vi "HandleObservationSync_003.vi"(8 "error in (no error)":errorcluster, 11 "S4GUI in":refnum<class "S4GUI.lvclass">) -> (0 "error out":errorcluster, 3 "S4GUI out":refnum<class "S4GUI.lvclass">)   [LabVIEW 2018, in "S4GUI.lvclass"]
uses:
  S4GUI.lvclass
  S4GUI.lvclass/S4GUI.ctl
  Instrument/Instrument.lvclass/Instrument.ctl
  Device/Optics/Optics.lvclass/Optics.ctl
  Server/Server.lvclass/Server.ctl
  Interface/Interface.lvclass/Interface.ctl
  Device/Optics/Opt_Selector/Opt_Selector.lvclass
  C:/Users/devstaff/sparc4/s4gui/Versao ZeroMQ REQ-REP/SPARC4_GUI -20241016_20241016/Device/Optics/Optics.lvclass
  Acquisition/Acquisition.lvclass
  C:/Users/devstaff/sparc4/s4gui/Versao ZeroMQ REQ-REP/SPARC4_GUI -20241016_20241016/Server/Server.lvclass
  SyncBox/Sync Box.lvclass
  Instrument/Instrument.lvclass
  Device/Optics/Opt_Continuous/Opt_Continuous.lvclass
  StateMachine/State Machine.lvclass
  Trigger/Trigger.lvclass
  Channel/Channel.lvclass
  Interface/Interface.lvclass
  TelFocus/TelFocus.lvclass
  SecMirror/SecMirror.lvclass
  Device/Optics/Optics.lvclass
  Server/Server.lvclass
panel:
  out "time1 3":u32
  out "time307":u32
  out "time9":u32
  out "time 10":u32
  out "delay 89":u32
  out "time1 2":u32
  out "delay Acq 2":u32
  out "time 8":u32
  out "delay 78":u32
  out "time elapsed 2":u32
  out "time7":u32
  out "time6":u32
  out "time5":u32
  out "time elapsed":u32
  out "timer351":u32
  out "delay wp 2":u32
  out "timer350":u32
  out "delay Acq":u32
  out "time308":u32
  out "delay wp":u32
  out "delay 3-4":u32
  out "time4":u32
  out "time3":u32
  out "time 2":u32
  out "time1":u32
  # "WAVEPLATE DURATION"
  # "ACS SETUP"
  # "Waveplate Test"
  # "Focus sequence"
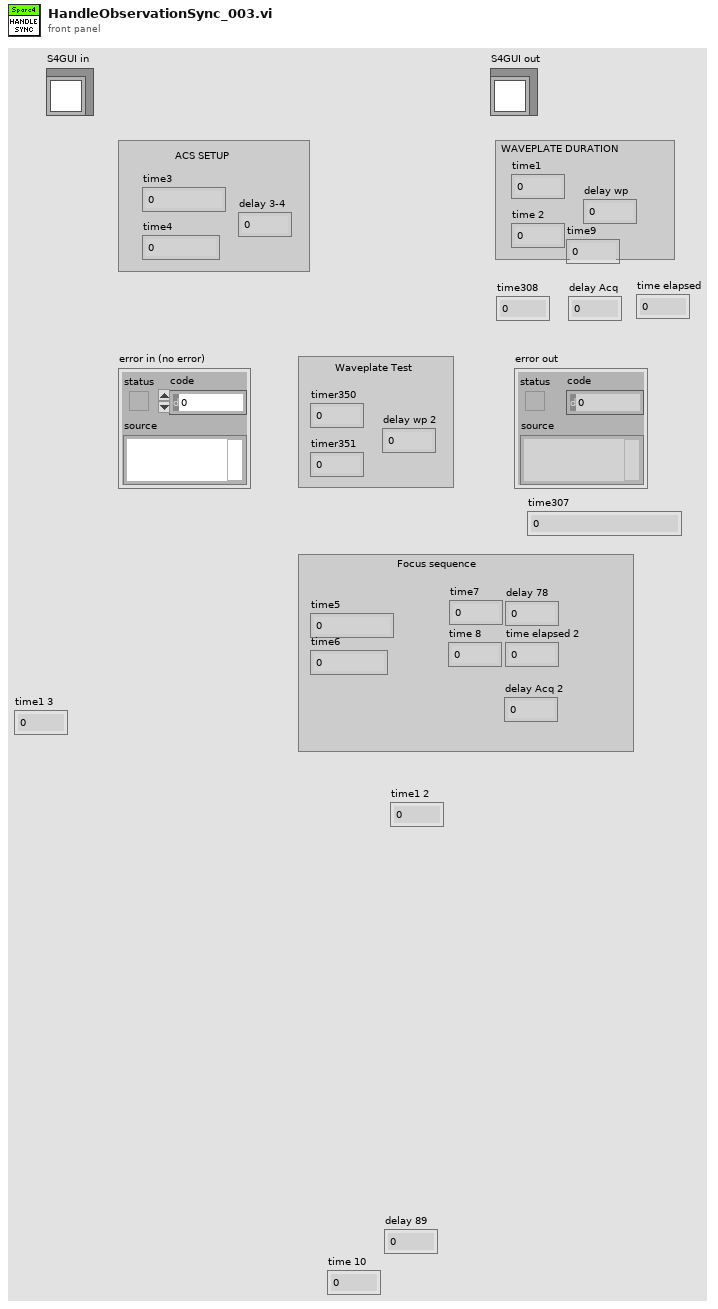
[diagram p1: front panel]
types:
  T1 = cluster{"ACQUISITION_MODE":u8, "TRIGGER_MODE":u8, "READ_MODE":u8, "PREAMP":u8, "READOUT_RATE":u8, "VERTICAL_SHIFT_SPEED":u8, "EM_MODE":u8, "EM_GAIN":u16, "SHUTTER_MODE":u8, "SHUTTER_TTL":u8, "SHUTTER_OPENING_TIME":u16, "SHUTTER_CLOSING_TIME":u16, "VBIN":u16, "HBIN":u16, "INITIAL_LINE":u16, "INITIAL_COLUMN":u16, "FINAL_LINE":u16, "FINAL_COLUMN":u16, "FRAME_TRANSFER":bool, "VERTICAL_CLOCK_VOLTAGE":u8, "AD_CHANNEL":u32}
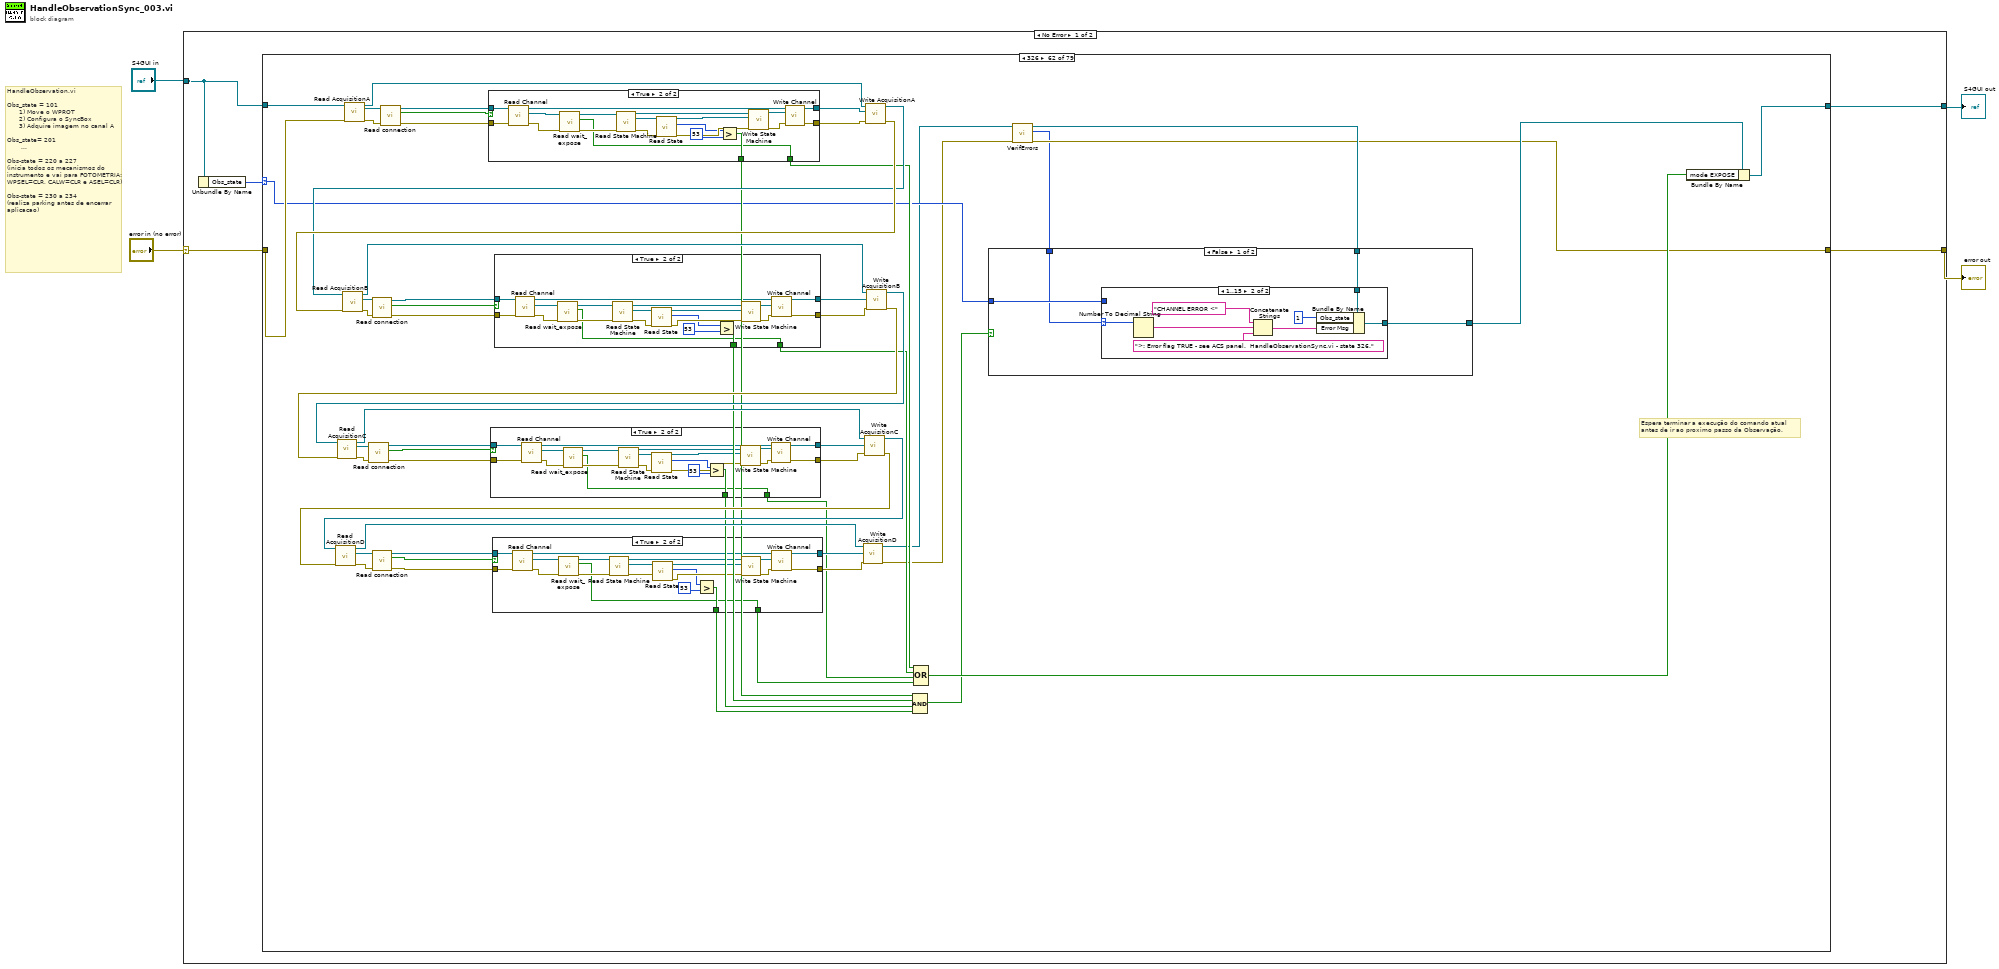
[diagram p0: block diagram]
diagram:
  # "HandleObservation.vi\n\nObs_state = 101\n      1) Move o WPROT\n      2) Configura o SyncBox\n      3) Adquire imagem no canal A\n\nObs_state= 201\n       ...\n\nObs-state = 220 a 227 \n(inicia todos os mecanismos do instrumento e vai para FOTOMETRIA: WPSEL=CLR, CALW=CLR e ASEL=CLR)\n\nObs-state = 230 a 234 \n(realiza parking antes de encerrar aplicacao)"
  n1 = case shown="No Error" "error in (no error)" {
    selector: "error in (no error)" -> [w8 w5859]
    tunnel: [w7 w5859] -> w3
    tunnel: [w9 w5858] -> w2
    tunnel: "S4GUI in" -> [w6 w5858]
    frame No Error {
      n2 = Unbundle By Name(w6) -> ("Obs_state"=w5:u32)
      n3 = case shown="326" w5 {
        selector: w5 -> [_ _ w18 w40 w66 w88 w114 w136 w204 w267 w292 w314 w340 w362 w397 w410 w432 w494 w526 w565 w611 w691 w723 w795 w804 w843 w854 _ w927 w1094 w1306 w1309 w1344 w1380 w1452 w1456 w1487 w1523 w1595 w1599 w1630 w1662 w1732 w1736 w1802 w1907 w2050 _ w2257 w2432 w2475 w2534 w2603 _ w3006 _ w3273 w3448 w3485 w3653 w3843 w4077 w4247 w4534 w4705 w4776 w4821 _ w4907 w4947 w5017 w5105 w5245 w5293 w5380 w5519 _ _ _]
        tunnel: w6 -> [w12 w14 w32 w57 w80 w105 w128 w153 w218 w285 w306 w331 w354 w379 w401 w424 w449 w503 w534 w571 w615 w700 w731 w801 w838 w847 w857 w865 w931 w1133 w1299 w1327 w1348 w1397 w1445 w1473 w1491 w1540 w1588 w1616 w1634 w1679 w1725 w1753 w1807 w1953 w2066 w2223 w2292 w2429 w2478 w2556 w2638 w2770 w3030 w3235 w3308 w3445 w3520 w3700 w3842 w4125 w4272 w4500 w4709 w4779 w4839 w4853 w4910 w4958 w5019 w5144 w5243 w5295 w5419 w5554 w5831 w5838 w5845]
        tunnel: [w10 w14 w16 w44 w64 w96 w112 w144 w202 w272 w290 w318 w338 w366 w396 w408 w436 w498 w528 w566 w613 w695 w725 w796 w832 w845 w855 w863 w930 w1093 w1304 w1318 w1342 w1388 w1450 w1464 w1485 w1531 w1593 w1607 w1628 w1670 w1730 w1744 w1767 w1906 w2052 w2222 w2290 w2437 w2473 w2539 w2636 w2829 w3007 w3243 w3306 w3453 w3518 w3698 w3844 w4123 w4245 w4535 w4706 w4774 w4824 w4850 w4905 w4949 w5015 w5142 w5247 w5291 w5417 w5588 w5836 w5838 w5842] -> w9
        tunnel: w8 -> [w13 w15 w31 w56 w79 w104 w127 w152 w217 w284 w305 w330 w353 w378 w400 w423 w448 w502 w533 w570 w614 w699 w730 w800 w837 w846 w856 w864 w914 w1124 w1300 w1326 w1347 w1396 w1446 w1472 w1490 w1539 w1589 w1615 w1633 w1678 w1726 w1752 w1786 w1943 w2100 w2213 w2291 w2430 w2443 w2549 w2637 w2830 w3064 w3244 w3307 w3446 w3519 w3699 w3847 w4124 w4305 w4536 w4708 w4744 w4830 w4852 w4899 w4954 w5018 w5143 w5242 w5294 w5418 w5589 w5827 w5837 w5841]
        tunnel: [w13 w15 w30 w55 w78 w103 w126 w151 w216 w283 w304 w329 w352 w377 w399 w422 w447 w501 w507 w569 w592 w698 w705 w799 w813 w846 w856 w864 w916 w1080 w1297 w1325 w1346 w1395 w1443 w1471 w1489 w1538 w1586 w1614 w1632 w1677 w1723 w1751 w1760 w1944 w2083 w2214 w2274 w2435 w2477 w2537 w2620 w2782 w3047 w3244 w3290 w3451 w3502 w3646 w3846 w4072 w4289 w4517 w4707 w4778 w4820 w4851 w4909 w4948 w4977 w5094 w5241 w5275 w5374 w5571 w5826 w5837 w5839] -> w7
        frame 0, Default {
          # "Nenhuma observação em andamento."
          n4 = Bundle By Name(cluster=w12, "Obs_state"=u32 0) -> (w10:refnum<class "S4GUI.lvclass">)
        }
        frame 1 {
          # "Estado de erro!\nFica aqui até acionar STOP ou ABORT."
          # "Nenhuma observação em andamento."
        }
        frame 101 {
          # "Dispara o comando para o dispositivo corrente."
          n5 = call "Read Instrument.lvclass.vi"("error in (no error)"=w31, "S4ACS_GUI in"=w32) -> ("error out"=w37:errorcluster, "Instrument.lvclass"=w38:refnum<class "Instrument.lvclass">, "S4ACS_GUI out"=w34:refnum<class "S4GUI.lvclass">)  [unwired: 7 in]
          n6 = call "Read WPROT.vi"("error in (no error)"=w37, "Instrument in"=w38) -> ("error out"=w24:errorcluster, "Opt_Selector.lvclass"=w23:refnum<class "Opt_Selector.lvclass">, "Instrument out"=w36:refnum<class "Instrument.lvclass">)  [unwired: 7 in]
          n7 = call-dynamic "Read State Machine.vi"("error in (no error)"=w24, "Device in"=w23) -> ("error out"=w27:errorcluster, "State Machine.lvclass"=w29:refnum<class "State Machine.lvclass">, "Device out"=w21:refnum<class "Opt_Selector.lvclass">)  [unwired: 7 in]
          n8 = call "Next State.vi"("error in (no error)"=w27, "New_State"=1, "State Machine in"=w29) -> ("error out"=w26:errorcluster, "State Machine out"=w25:refnum<class "State Machine.lvclass">)  [unwired: 7 in]
          n9 = call-dynamic "Write State Machine.vi"("error in (no error)"=w26, "State Machine.lvclass"=w25, "Device in"=w21) -> ("error out"=w20:errorcluster, "Device out"=w22:refnum<class "Opt_Selector.lvclass">)  [unwired: 7 in]
          n10 = Increment(x=w18) -> (x+1=w17:u32)
          n11 = call "Write WPROT.vi"("error in (no error)"=w20, "Opt_Selector.lvclass"=w22, "Instrument in"=w36) -> ("error out"=w33:errorcluster, "Instrument out"=w35:refnum<class "Instrument.lvclass">)  [unwired: 7 in]
          n12 = call "Write Instrument.lvclass.vi"("error in (no error)"=w33, "Instrument.lvclass"=w35, "S4ACS_GUI in"=w34) -> ("error out"=w30:errorcluster, "S4ACS_GUI out"=w19:refnum<class "S4GUI.lvclass">)  [unwired: 7 in]
          n13 = Bundle By Name(cluster=w19, "Obs_state"=w17) -> (w16:refnum<class "S4GUI.lvclass">)
        }
        frame 102 {
          # "Espera terminar a execução do comando atual \nantes de ir ao proximo passo da Observação."
          n14 = call "Read Instrument.lvclass.vi"("error in (no error)"=w56, "S4ACS_GUI in"=w57) -> ("error out"=w62:errorcluster, "Instrument.lvclass"=w63:refnum<class "Instrument.lvclass">, "S4ACS_GUI out"=w59:refnum<class "S4GUI.lvclass">)  [unwired: 7 in]
          n15 = call "Read WPROT.vi"("error in (no error)"=w62, "Instrument in"=w63) -> ("error out"=w50:errorcluster, "Opt_Selector.lvclass"=w49:refnum<class "Opt_Selector.lvclass">, "Instrument out"=w61:refnum<class "Instrument.lvclass">)  [unwired: 7 in]
          n16 = call-dynamic "Read State Machine.vi"("error in (no error)"=w50, "Device in"=w49) -> ("error out"=w53:errorcluster, "State Machine.lvclass"=w54:refnum<class "State Machine.lvclass">, "Device out"=w47:refnum<class "Opt_Selector.lvclass">)  [unwired: 7 in]
          n17 = Increment(x=w40) -> (x+1=w39:u32)
          n18 = call-dynamic "Read State.vi"("error in (no error)"=w53, "State Machine in"=w54) -> ("error out"=w52:errorcluster, "State"=w42:i32, "State Machine out"=w51:refnum<class "State Machine.lvclass">)  [unwired: 7 in]
          n19 = Equal To 0?(x=w42) -> (x = 0?=w43:bool)
          n20 = call-dynamic "Write State Machine.vi"("error in (no error)"=w52, "State Machine.lvclass"=w51, "Device in"=w47) -> ("error out"=w46:errorcluster, "Device out"=w48:refnum<class "Opt_Selector.lvclass">)  [unwired: 7 in]
          n21 = call "Write WPROT.vi"("error in (no error)"=w46, "Opt_Selector.lvclass"=w48, "Instrument in"=w61) -> ("error out"=w58:errorcluster, "Instrument out"=w60:refnum<class "Instrument.lvclass">)  [unwired: 7 in]
          n22 = Select(t=w39, s=w43, f=w40) -> (s? t:f=w41:u32)
          n23 = call "Write Instrument.lvclass.vi"("error in (no error)"=w58, "Instrument.lvclass"=w60, "S4ACS_GUI in"=w59) -> ("error out"=w55:errorcluster, "S4ACS_GUI out"=w45:refnum<class "S4GUI.lvclass">)  [unwired: 7 in]
          n24 = Bundle By Name(cluster=w45, "Obs_state"=w41) -> (w44:refnum<class "S4GUI.lvclass">)
        }
        frame 103 {
          # "Dispara o comando para o dispositivo corrente."
          n25 = call-dynamic "Read Sync Box.lvclass.vi"("error in (no error)"=w79, "SPARC4_AC in"=w80) -> ("error out"=w85:errorcluster, "Sync Box.lvclass"=w86:refnum<class "Sync Box.lvclass">, "SPARC4_AC out"=w82:refnum<class "S4GUI.lvclass">)  [unwired: 7 in]
          n26 = call-dynamic "Read Trigger.lvclass.vi"("error in (no error)"=w85, "Sync Box in"=w86) -> ("error out"=w72:errorcluster, "Trigger.lvclass"=w71:refnum<class "Trigger.lvclass">, "Sync Box out"=w84:refnum<class "Sync Box.lvclass">)  [unwired: 7 in]
          n27 = call-dynamic "Read State Machine.vi"("error in (no error)"=w72, "Device in"=w71) -> ("error out"=w75:errorcluster, "State Machine.lvclass"=w77:refnum<class "State Machine.lvclass">, "Device out"=w69:refnum<class "Trigger.lvclass">)  [unwired: 7 in]
          n28 = call "Next State.vi"("error in (no error)"=w75, "New_State"=1, "State Machine in"=w77) -> ("error out"=w74:errorcluster, "State Machine out"=w73:refnum<class "State Machine.lvclass">)  [unwired: 7 in]
          n29 = call-dynamic "Write State Machine.vi"("error in (no error)"=w74, "State Machine.lvclass"=w73, "Device in"=w69) -> ("error out"=w68:errorcluster, "Device out"=w70:refnum<class "Trigger.lvclass">)  [unwired: 7 in]
          n30 = Increment(x=w66) -> (x+1=w65:u32)
          n31 = call-dynamic "Write Trigger.lvclass.vi"("error in (no error)"=w68, "Trigger.lvclass"=w70, "Sync Box in"=w84) -> ("error out"=w81:errorcluster, "Sync Box out"=w83:refnum<class "Sync Box.lvclass">)  [unwired: 7 in]
          n32 = call-dynamic "Write Sync Box.lvclass.vi"("error in (no error)"=w81, "Sync Box.lvclass"=w83, "SPARC4_AC in"=w82) -> ("error out"=w78:errorcluster, "SPARC4_AC out"=w67:refnum<class "S4GUI.lvclass">)  [unwired: 7 in]
          n33 = Bundle By Name(cluster=w67, "Obs_state"=w65) -> (w64:refnum<class "S4GUI.lvclass">)
        }
        frame 104 {
          # "Espera terminar a execução do comando atual \nantes de ir ao proximo passo da Observação."
          n34 = call-dynamic "Read Sync Box.lvclass.vi"("error in (no error)"=w104, "SPARC4_AC in"=w105) -> ("error out"=w110:errorcluster, "Sync Box.lvclass"=w111:refnum<class "Sync Box.lvclass">, "SPARC4_AC out"=w107:refnum<class "S4GUI.lvclass">)  [unwired: 7 in]
          n35 = call-dynamic "Read Trigger.lvclass.vi"("error in (no error)"=w110, "Sync Box in"=w111) -> ("error out"=w102:errorcluster, "Trigger.lvclass"=w101:refnum<class "Trigger.lvclass">, "Sync Box out"=w109:refnum<class "Sync Box.lvclass">)  [unwired: 7 in]
          n36 = call-dynamic "Read State Machine.vi"("error in (no error)"=w102, "Device in"=w101) -> ("error out"=w93:errorcluster, "State Machine.lvclass"=w95:refnum<class "State Machine.lvclass">, "Device out"=w99:refnum<class "Trigger.lvclass">)  [unwired: 7 in]
          n37 = Increment(x=w88) -> (x+1=w90:u32)
          n38 = call-dynamic "Read State.vi"("error in (no error)"=w93, "State Machine in"=w95) -> ("error out"=w92:errorcluster, "State"=w87:i32, "State Machine out"=w94:refnum<class "State Machine.lvclass">)  [unwired: 7 in]
          n39 = Equal To 0?(x=w87) -> (x = 0?=w91:bool)
          n40 = call-dynamic "Write State Machine.vi"("error in (no error)"=w92, "State Machine.lvclass"=w94, "Device in"=w99) -> ("error out"=w98:errorcluster, "Device out"=w100:refnum<class "Trigger.lvclass">)  [unwired: 7 in]
          n41 = call-dynamic "Write Trigger.lvclass.vi"("error in (no error)"=w98, "Trigger.lvclass"=w100, "Sync Box in"=w109) -> ("error out"=w106:errorcluster, "Sync Box out"=w108:refnum<class "Sync Box.lvclass">)  [unwired: 7 in]
          n42 = Select(t=w90, s=w91, f=w88) -> (s? t:f=w89:u32)
          n43 = call-dynamic "Write Sync Box.lvclass.vi"("error in (no error)"=w106, "Sync Box.lvclass"=w108, "SPARC4_AC in"=w107) -> ("error out"=w103:errorcluster, "SPARC4_AC out"=w97:refnum<class "S4GUI.lvclass">)  [unwired: 7 in]
          n44 = Bundle By Name(cluster=w97, "Obs_state"=w89) -> (w96:refnum<class "S4GUI.lvclass">)
        }
        frame 105 {
          # "Dispara o comando para o dispositivo corrente."
          n45 = call-dynamic "Read AcquisitionA.vi"("error in (no error)"=w127, "S4ACS_GUI in"=w128) -> ("error out"=w133:errorcluster, "Acquisition.lvclass"=w134:refnum<class "Acquisition.lvclass">, "S4ACS_GUI out"=w130:refnum<class "S4GUI.lvclass">)  [unwired: 7 in]
          n46 = call-dynamic "Read Channel.vi"("error in (no error)"=w133, "Acquisition in"=w134) -> ("error out"=w120:errorcluster, "Channel.lvclass"=w119:refnum<class "Channel.lvclass">, "Acquisition out"=w132:refnum<class "Acquisition.lvclass">)  [unwired: 7 in]
          n47 = call-dynamic "Read State Machine.vi"("error in (no error)"=w120, "Device in"=w119) -> ("error out"=w123:errorcluster, "State Machine.lvclass"=w125:refnum<class "State Machine.lvclass">, "Device out"=w117:refnum<class "Channel.lvclass">)  [unwired: 7 in]
          n48 = call "Next State.vi"("error in (no error)"=w123, "New_State"=1, "State Machine in"=w125) -> ("error out"=w122:errorcluster, "State Machine out"=w121:refnum<class "State Machine.lvclass">)  [unwired: 7 in]
          n49 = call-dynamic "Write State Machine.vi"("error in (no error)"=w122, "State Machine.lvclass"=w121, "Device in"=w117) -> ("error out"=w116:errorcluster, "Device out"=w118:refnum<class "Channel.lvclass">)  [unwired: 7 in]
          n50 = Increment(x=w114) -> (x+1=w113:u32)
          n51 = call-dynamic "Write Channel.vi"("error in (no error)"=w116, "Channel.lvclass"=w118, "Acquisition in"=w132) -> ("error out"=w129:errorcluster, "Acquisition out"=w131:refnum<class "Acquisition.lvclass">)  [unwired: 7 in]
          n52 = call-dynamic "Write AcquisitionA.vi"("error in (no error)"=w129, "Acquisition.lvclass"=w131, "S4ACS_GUI in"=w130) -> ("error out"=w126:errorcluster, "S4ACS_GUI out"=w115:refnum<class "S4GUI.lvclass">)  [unwired: 7 in]
          n53 = Bundle By Name(cluster=w115, "Obs_state"=w113) -> (w112:refnum<class "S4GUI.lvclass">)
        }
        frame 106 {
          # "Espera terminar a execução do comando atual \nantes de ir ao proximo passo da Observação."
          n54 = call-dynamic "Read AcquisitionA.vi"("error in (no error)"=w152, "S4ACS_GUI in"=w153) -> ("error out"=w158:errorcluster, "Acquisition.lvclass"=w159:refnum<class "Acquisition.lvclass">, "S4ACS_GUI out"=w155:refnum<class "S4GUI.lvclass">)  [unwired: 7 in]
          n55 = call-dynamic "Read Channel.vi"("error in (no error)"=w158, "Acquisition in"=w159) -> ("error out"=w150:errorcluster, "Channel.lvclass"=w149:refnum<class "Channel.lvclass">, "Acquisition out"=w157:refnum<class "Acquisition.lvclass">)  [unwired: 7 in]
          n56 = call-dynamic "Read State Machine.vi"("error in (no error)"=w150, "Device in"=w149) -> ("error out"=w141:errorcluster, "State Machine.lvclass"=w143:refnum<class "State Machine.lvclass">, "Device out"=w147:refnum<class "Channel.lvclass">)  [unwired: 7 in]
          n57 = Increment(x=w136) -> (x+1=w138:u32)
          n58 = call-dynamic "Read State.vi"("error in (no error)"=w141, "State Machine in"=w143) -> ("error out"=w140:errorcluster, "State"=w135:i32, "State Machine out"=w142:refnum<class "State Machine.lvclass">)  [unwired: 7 in]
          n59 = Equal To 0?(x=w135) -> (x = 0?=w139:bool)
          n60 = call-dynamic "Write State Machine.vi"("error in (no error)"=w140, "State Machine.lvclass"=w142, "Device in"=w147) -> ("error out"=w146:errorcluster, "Device out"=w148:refnum<class "Channel.lvclass">)  [unwired: 7 in]
          n61 = call-dynamic "Write Channel.vi"("error in (no error)"=w146, "Channel.lvclass"=w148, "Acquisition in"=w157) -> ("error out"=w154:errorcluster, "Acquisition out"=w156:refnum<class "Acquisition.lvclass">)  [unwired: 7 in]
          n62 = Select(t=w138, s=w139, f=w136) -> (s? t:f=w137:u32)
          n63 = call-dynamic "Write AcquisitionA.vi"("error in (no error)"=w154, "Acquisition.lvclass"=w156, "S4ACS_GUI in"=w155) -> ("error out"=w151:errorcluster, "S4ACS_GUI out"=w145:refnum<class "S4GUI.lvclass">)  [unwired: 7 in]
          n64 = Bundle By Name(cluster=w145, "Obs_state"=w137) -> (w144:refnum<class "S4GUI.lvclass">)
        }
        frame 200 {
          # "Seleção do MODO DE OPERAÇÃO (configurar ASEL, CALW, WPSEL e WPROT): \nFotometria; Polarimetria Linear; Polarimetria Circular; Eficiencia de Polar. Linear; Eficiencia de Polar. Circular;\nPolarizacao Linear Instrumental e POolarização Circular Instrumental."
          n65 = call "Read Instrument.lvclass.vi"("error in (no error)"=w217, "S4ACS_GUI in"=w218) -> ("error out"=w221:errorcluster, "Instrument.lvclass"=w181:refnum<class "Instrument.lvclass">, "S4ACS_GUI out"=w219:refnum<class "S4GUI.lvclass">)  [unwired: 7 in]
          n66 = call "Read ASEL.vi"("error in (no error)"=w221, "Instrument in"=w181) -> ("error out"=w210:errorcluster, "Opt_Selector.lvclass"=w209:refnum<class "Opt_Selector.lvclass">, "Instrument out"=w220:refnum<class "Instrument.lvclass">)  [unwired: 7 in]
          n67 = call-dynamic "Read State Machine.vi"("error in (no error)"=w210, "Device in"=w209) -> ("error out"=w213:errorcluster, "State Machine.lvclass"=w215:refnum<class "State Machine.lvclass">, "Device out"=w207:refnum<class "Opt_Selector.lvclass">)  [unwired: 7 in]
          n68 = call "Next State.vi"("error in (no error)"=w213, "New_State"=1, "State Machine in"=w215) -> ("error out"=w212:errorcluster, "State Machine out"=w211:refnum<class "State Machine.lvclass">)  [unwired: 7 in]
          n69 = call-dynamic "Write State Machine.vi"("error in (no error)"=w212, "State Machine.lvclass"=w211, "Device in"=w207) -> ("error out"=w206:errorcluster, "Device out"=w208:refnum<class "Opt_Selector.lvclass">)  [unwired: 7 in]
          n70 = Increment(x=w204) -> (x+1=w203:u32)
          n71 = call "Write ASEL.vi"("error in (no error)"=w206, "Opt_Selector.lvclass"=w208, "Instrument in"=w220) -> ("error out"=w162:errorcluster, "Instrument out"=w180:refnum<class "Instrument.lvclass">)  [unwired: 7 in]
          n72 = call "Read CALW.vi"("error in (no error)"=w162, "Instrument in"=w180) -> ("error out"=w197:errorcluster, "Opt_Selector.lvclass"=w198:refnum<class "Opt_Selector.lvclass">, "Instrument out"=w179:refnum<class "Instrument.lvclass">)  [unwired: 7 in]
          n73 = call-dynamic "Read State Machine.vi"("error in (no error)"=w197, "Device in"=w198) -> ("error out"=w194:errorcluster, "State Machine.lvclass"=w192:refnum<class "State Machine.lvclass">, "Device out"=w200:refnum<class "Opt_Selector.lvclass">)  [unwired: 7 in]
          n74 = call "Next State.vi"("error in (no error)"=w194, "New_State"=1, "State Machine in"=w192) -> ("error out"=w195:errorcluster, "State Machine out"=w196:refnum<class "State Machine.lvclass">)  [unwired: 7 in]
          n75 = call-dynamic "Write State Machine.vi"("error in (no error)"=w195, "State Machine.lvclass"=w196, "Device in"=w200) -> ("error out"=w201:errorcluster, "Device out"=w199:refnum<class "Opt_Selector.lvclass">)  [unwired: 7 in]
          n76 = call "Write CALW.vi"("error in (no error)"=w201, "Opt_Selector.lvclass"=w199, "Instrument in"=w179) -> ("error out"=w161:errorcluster, "Instrument out"=w178:refnum<class "Instrument.lvclass">)  [unwired: 7 in]
          n77 = call "Read WPSEL.vi"("error in (no error)"=w161, "Instrument in"=w178) -> ("error out"=w186:errorcluster, "Opt_Selector.lvclass"=w185:refnum<class "Opt_Selector.lvclass">, "Instrument out"=w177:refnum<class "Instrument.lvclass">)  [unwired: 7 in]
          n78 = call-dynamic "Read State Machine.vi"("error in (no error)"=w186, "Device in"=w185) -> ("error out"=w189:errorcluster, "State Machine.lvclass"=w191:refnum<class "State Machine.lvclass">, "Device out"=w183:refnum<class "Opt_Selector.lvclass">)  [unwired: 7 in]
          n79 = call "Next State.vi"("error in (no error)"=w189, "New_State"=1, "State Machine in"=w191) -> ("error out"=w188:errorcluster, "State Machine out"=w187:refnum<class "State Machine.lvclass">)  [unwired: 7 in]
          n80 = call-dynamic "Write State Machine.vi"("error in (no error)"=w188, "State Machine.lvclass"=w187, "Device in"=w183) -> ("error out"=w182:errorcluster, "Device out"=w184:refnum<class "Opt_Selector.lvclass">)  [unwired: 7 in]
          n81 = call "Write WPSEL.vi"("error in (no error)"=w182, "Opt_Selector.lvclass"=w184, "Instrument in"=w177) -> ("error out"=w160:errorcluster, "Instrument out"=w166:refnum<class "Instrument.lvclass">)  [unwired: 7 in]
          n82 = call "Read WPROT.vi"("error in (no error)"=w160, "Instrument in"=w166) -> ("error out"=w172:errorcluster, "Opt_Selector.lvclass"=w173:refnum<class "Opt_Selector.lvclass">, "Instrument out"=w165:refnum<class "Instrument.lvclass">)  [unwired: 7 in]
          n83 = call-dynamic "Read State Machine.vi"("error in (no error)"=w172, "Device in"=w173) -> ("error out"=w169:errorcluster, "State Machine.lvclass"=w167:refnum<class "State Machine.lvclass">, "Device out"=w175:refnum<class "Opt_Selector.lvclass">)  [unwired: 7 in]
          n84 = call "Next State.vi"("error in (no error)"=w169, "New_State"=1, "State Machine in"=w167) -> ("error out"=w170:errorcluster, "State Machine out"=w171:refnum<class "State Machine.lvclass">)  [unwired: 7 in]
          n85 = call-dynamic "Write State Machine.vi"("error in (no error)"=w170, "State Machine.lvclass"=w171, "Device in"=w175) -> ("error out"=w176:errorcluster, "Device out"=w174:refnum<class "Opt_Selector.lvclass">)  [unwired: 7 in]
          n86 = call "Write WPROT.vi"("error in (no error)"=w176, "Opt_Selector.lvclass"=w174, "Instrument in"=w165) -> ("error out"=w163:errorcluster, "Instrument out"=w164:refnum<class "Instrument.lvclass">)  [unwired: 7 in]
          n87 = call "Write Instrument.lvclass.vi"("error in (no error)"=w163, "Instrument.lvclass"=w164, "S4ACS_GUI in"=w219) -> ("error out"=w216:errorcluster, "S4ACS_GUI out"=w205:refnum<class "S4GUI.lvclass">)  [unwired: 7 in]
          n88 = Bundle By Name(cluster=w205, "Obs_state"=w203) -> (w202:refnum<class "S4GUI.lvclass">)
        }
        frame 201 {
          # "Espera terminar a execução dos comandos ."
          n89 = call "Read Instrument.lvclass.vi"("error in (no error)"=w284, "S4ACS_GUI in"=w285) -> ("error out"=w288:errorcluster, "Instrument.lvclass"=w289:refnum<class "Instrument.lvclass">, "S4ACS_GUI out"=w286:refnum<class "S4GUI.lvclass">)  [unwired: 7 in]
          n90 = call "Read ASEL.vi"("error in (no error)"=w288, "Instrument in"=w289) -> ("error out"=w278:errorcluster, "Opt_Selector.lvclass"=w277:refnum<class "Opt_Selector.lvclass">, "Instrument out"=w287:refnum<class "Instrument.lvclass">)  [unwired: 7 in]
          n91 = call-dynamic "Read State Machine.vi"("error in (no error)"=w278, "Device in"=w277) -> ("error out"=w281:errorcluster, "State Machine.lvclass"=w282:refnum<class "State Machine.lvclass">, "Device out"=w275:refnum<class "Opt_Selector.lvclass">)  [unwired: 7 in]
          n92 = call-dynamic "Read State.vi"("error in (no error)"=w281, "State Machine in"=w282) -> ("error out"=w280:errorcluster, "State"=w271:i32, "State Machine out"=w279:refnum<class "State Machine.lvclass">)  [unwired: 7 in]
          n93 = Equal To 0?(x=w271) -> (x = 0?=w266:bool)
          n94 = call-dynamic "Write State Machine.vi"("error in (no error)"=w280, "State Machine.lvclass"=w279, "Device in"=w275) -> ("error out"=w274:errorcluster, "Device out"=w276:refnum<class "Opt_Selector.lvclass">)  [unwired: 7 in]
          n95 = call "Write ASEL.vi"("error in (no error)"=w274, "Opt_Selector.lvclass"=w276, "Instrument in"=w287) -> ("error out"=w228:errorcluster, "Instrument out"=w229:refnum<class "Instrument.lvclass">)  [unwired: 7 in]
          n96 = call "Read CALW.vi"("error in (no error)"=w228, "Instrument in"=w229) -> ("error out"=w261:errorcluster, "Opt_Selector.lvclass"=w262:refnum<class "Opt_Selector.lvclass">, "Instrument out"=w232:refnum<class "Instrument.lvclass">)  [unwired: 7 in]
          n97 = call-dynamic "Read State Machine.vi"("error in (no error)"=w261, "Device in"=w262) -> ("error out"=w258:errorcluster, "State Machine.lvclass"=w257:refnum<class "State Machine.lvclass">, "Device out"=w264:refnum<class "Opt_Selector.lvclass">)  [unwired: 7 in]
          n98 = call-dynamic "Read State.vi"("error in (no error)"=w258, "State Machine in"=w257) -> ("error out"=w259:errorcluster, "State"=w256:i32, "State Machine out"=w260:refnum<class "State Machine.lvclass">)  [unwired: 7 in]
          n99 = Equal To 0?(x=w256) -> (x = 0?=w255:bool)
          n100 = call-dynamic "Write State Machine.vi"("error in (no error)"=w259, "State Machine.lvclass"=w260, "Device in"=w264) -> ("error out"=w265:errorcluster, "Device out"=w263:refnum<class "Opt_Selector.lvclass">)  [unwired: 7 in]
          n101 = call "Write CALW.vi"("error in (no error)"=w265, "Opt_Selector.lvclass"=w263, "Instrument in"=w232) -> ("error out"=w226:errorcluster, "Instrument out"=w227:refnum<class "Instrument.lvclass">)  [unwired: 7 in]
          n102 = call "Read WPSEL.vi"("error in (no error)"=w226, "Instrument in"=w227) -> ("error out"=w249:errorcluster, "Opt_Selector.lvclass"=w248:refnum<class "Opt_Selector.lvclass">, "Instrument out"=w231:refnum<class "Instrument.lvclass">)  [unwired: 7 in]
          n103 = call-dynamic "Read State Machine.vi"("error in (no error)"=w249, "Device in"=w248) -> ("error out"=w252:errorcluster, "State Machine.lvclass"=w253:refnum<class "State Machine.lvclass">, "Device out"=w246:refnum<class "Opt_Selector.lvclass">)  [unwired: 7 in]
          n104 = call-dynamic "Read State.vi"("error in (no error)"=w252, "State Machine in"=w253) -> ("error out"=w251:errorcluster, "State"=w254:i32, "State Machine out"=w250:refnum<class "State Machine.lvclass">)  [unwired: 7 in]
          n105 = Equal To 0?(x=w254) -> (x = 0?=w234:bool)
          n106 = call-dynamic "Write State Machine.vi"("error in (no error)"=w251, "State Machine.lvclass"=w250, "Device in"=w246) -> ("error out"=w245:errorcluster, "Device out"=w247:refnum<class "Opt_Selector.lvclass">)  [unwired: 7 in]
          n107 = call "Write WPSEL.vi"("error in (no error)"=w245, "Opt_Selector.lvclass"=w247, "Instrument in"=w231) -> ("error out"=w224:errorcluster, "Instrument out"=w225:refnum<class "Instrument.lvclass">)  [unwired: 7 in]
          n108 = call "Read WPROT.vi"("error in (no error)"=w224, "Instrument in"=w225) -> ("error out"=w240:errorcluster, "Opt_Selector.lvclass"=w241:refnum<class "Opt_Selector.lvclass">, "Instrument out"=w230:refnum<class "Instrument.lvclass">)  [unwired: 7 in]
          n109 = call-dynamic "Read State Machine.vi"("error in (no error)"=w240, "Device in"=w241) -> ("error out"=w237:errorcluster, "State Machine.lvclass"=w236:refnum<class "State Machine.lvclass">, "Device out"=w243:refnum<class "Opt_Selector.lvclass">)  [unwired: 7 in]
          n110 = call-dynamic "Read State.vi"("error in (no error)"=w237, "State Machine in"=w236) -> ("error out"=w238:errorcluster, "State"=w235:i32, "State Machine out"=w239:refnum<class "State Machine.lvclass">)  [unwired: 7 in]
          n111 = Equal To 0?(x=w235) -> (x = 0?=w233:bool)
          n112 = call-dynamic "Write State Machine.vi"("error in (no error)"=w238, "State Machine.lvclass"=w239, "Device in"=w243) -> ("error out"=w244:errorcluster, "Device out"=w242:refnum<class "Opt_Selector.lvclass">)  [unwired: 7 in]
          n113 = call "Write WPROT.vi"("error in (no error)"=w244, "Opt_Selector.lvclass"=w242, "Instrument in"=w230) -> ("error out"=w222:errorcluster, "Instrument out"=w223:refnum<class "Instrument.lvclass">)  [unwired: 7 in]
          n114 = Compound Arithmetic op=AND(w266, w255, w234, w233) -> (w268:bool)
          n115 = Select(t=u32 0, s=w268, f=w267) -> (s? t:f=w270:u32)
          n116 = call "Write Instrument.lvclass.vi"("error in (no error)"=w222, "Instrument.lvclass"=w223, "S4ACS_GUI in"=w286) -> ("error out"=w283:errorcluster, "S4ACS_GUI out"=w273:refnum<class "S4GUI.lvclass">)  [unwired: 7 in]
          n117 = Bundle By Name(cluster=w273, "Obs_state"=w270) -> (w272:refnum<class "S4GUI.lvclass">)
        }
        frame 202 {
          # "Dispara o comando para o dispositivo corrente."
          n118 = call "Read Instrument.lvclass.vi"("error in (no error)"=w305, "S4ACS_GUI in"=w306) -> ("error out"=w311:errorcluster, "Instrument.lvclass"=w312:refnum<class "Instrument.lvclass">, "S4ACS_GUI out"=w308:refnum<class "S4GUI.lvclass">)  [unwired: 7 in]
          n119 = call "Read CALW.vi"("error in (no error)"=w311, "Instrument in"=w312) -> ("error out"=w298:errorcluster, "Opt_Selector.lvclass"=w297:refnum<class "Opt_Selector.lvclass">, "Instrument out"=w310:refnum<class "Instrument.lvclass">)  [unwired: 7 in]
          n120 = call-dynamic "Read State Machine.vi"("error in (no error)"=w298, "Device in"=w297) -> ("error out"=w301:errorcluster, "State Machine.lvclass"=w303:refnum<class "State Machine.lvclass">, "Device out"=w295:refnum<class "Opt_Selector.lvclass">)  [unwired: 7 in]
          n121 = call "Next State.vi"("error in (no error)"=w301, "New_State"=1, "State Machine in"=w303) -> ("error out"=w300:errorcluster, "State Machine out"=w299:refnum<class "State Machine.lvclass">)  [unwired: 7 in]
          n122 = call-dynamic "Write State Machine.vi"("error in (no error)"=w300, "State Machine.lvclass"=w299, "Device in"=w295) -> ("error out"=w294:errorcluster, "Device out"=w296:refnum<class "Opt_Selector.lvclass">)  [unwired: 7 in]
          n123 = Increment(x=w292) -> (x+1=w291:u32)
          n124 = call "Write CALW.vi"("error in (no error)"=w294, "Opt_Selector.lvclass"=w296, "Instrument in"=w310) -> ("error out"=w307:errorcluster, "Instrument out"=w309:refnum<class "Instrument.lvclass">)  [unwired: 7 in]
          n125 = call "Write Instrument.lvclass.vi"("error in (no error)"=w307, "Instrument.lvclass"=w309, "S4ACS_GUI in"=w308) -> ("error out"=w304:errorcluster, "S4ACS_GUI out"=w293:refnum<class "S4GUI.lvclass">)  [unwired: 7 in]
          n126 = Bundle By Name(cluster=w293, "Obs_state"=w291) -> (w290:refnum<class "S4GUI.lvclass">)
        }
        frame 203 {
          # "Espera terminar a execução do comando atual \nantes de ir ao proximo passo da Observação."
          n127 = call "Read Instrument.lvclass.vi"("error in (no error)"=w330, "S4ACS_GUI in"=w331) -> ("error out"=w336:errorcluster, "Instrument.lvclass"=w337:refnum<class "Instrument.lvclass">, "S4ACS_GUI out"=w333:refnum<class "S4GUI.lvclass">)  [unwired: 7 in]
          n128 = call "Read CALW.vi"("error in (no error)"=w336, "Instrument in"=w337) -> ("error out"=w324:errorcluster, "Opt_Selector.lvclass"=w323:refnum<class "Opt_Selector.lvclass">, "Instrument out"=w335:refnum<class "Instrument.lvclass">)  [unwired: 7 in]
          n129 = call-dynamic "Read State Machine.vi"("error in (no error)"=w324, "Device in"=w323) -> ("error out"=w327:errorcluster, "State Machine.lvclass"=w328:refnum<class "State Machine.lvclass">, "Device out"=w321:refnum<class "Opt_Selector.lvclass">)  [unwired: 7 in]
          n130 = Increment(x=w314) -> (x+1=w313:u32)
          n131 = call-dynamic "Read State.vi"("error in (no error)"=w327, "State Machine in"=w328) -> ("error out"=w326:errorcluster, "State"=w316:i32, "State Machine out"=w325:refnum<class "State Machine.lvclass">)  [unwired: 7 in]
          n132 = Equal To 0?(x=w316) -> (x = 0?=w317:bool)
          n133 = call-dynamic "Write State Machine.vi"("error in (no error)"=w326, "State Machine.lvclass"=w325, "Device in"=w321) -> ("error out"=w320:errorcluster, "Device out"=w322:refnum<class "Opt_Selector.lvclass">)  [unwired: 7 in]
          n134 = call "Write CALW.vi"("error in (no error)"=w320, "Opt_Selector.lvclass"=w322, "Instrument in"=w335) -> ("error out"=w332:errorcluster, "Instrument out"=w334:refnum<class "Instrument.lvclass">)  [unwired: 7 in]
          n135 = Select(t=w313, s=w317, f=w314) -> (s? t:f=w315:u32)
          n136 = call "Write Instrument.lvclass.vi"("error in (no error)"=w332, "Instrument.lvclass"=w334, "S4ACS_GUI in"=w333) -> ("error out"=w329:errorcluster, "S4ACS_GUI out"=w319:refnum<class "S4GUI.lvclass">)  [unwired: 7 in]
          n137 = Bundle By Name(cluster=w319, "Obs_state"=w315) -> (w318:refnum<class "S4GUI.lvclass">)
        }
        frame 204 {
          # "Dispara o comando para o dispositivo corrente."
          n138 = call "Read Instrument.lvclass.vi"("error in (no error)"=w353, "S4ACS_GUI in"=w354) -> ("error out"=w359:errorcluster, "Instrument.lvclass"=w360:refnum<class "Instrument.lvclass">, "S4ACS_GUI out"=w356:refnum<class "S4GUI.lvclass">)  [unwired: 7 in]
          n139 = call "Read WPSEL.vi"("error in (no error)"=w359, "Instrument in"=w360) -> ("error out"=w346:errorcluster, "Opt_Selector.lvclass"=w345:refnum<class "Opt_Selector.lvclass">, "Instrument out"=w358:refnum<class "Instrument.lvclass">)  [unwired: 7 in]
          n140 = call-dynamic "Read State Machine.vi"("error in (no error)"=w346, "Device in"=w345) -> ("error out"=w349:errorcluster, "State Machine.lvclass"=w351:refnum<class "State Machine.lvclass">, "Device out"=w343:refnum<class "Opt_Selector.lvclass">)  [unwired: 7 in]
          n141 = call "Next State.vi"("error in (no error)"=w349, "New_State"=1, "State Machine in"=w351) -> ("error out"=w348:errorcluster, "State Machine out"=w347:refnum<class "State Machine.lvclass">)  [unwired: 7 in]
          n142 = call-dynamic "Write State Machine.vi"("error in (no error)"=w348, "State Machine.lvclass"=w347, "Device in"=w343) -> ("error out"=w342:errorcluster, "Device out"=w344:refnum<class "Opt_Selector.lvclass">)  [unwired: 7 in]
          n143 = Increment(x=w340) -> (x+1=w339:u32)
          n144 = call "Write WPSEL.vi"("error in (no error)"=w342, "Opt_Selector.lvclass"=w344, "Instrument in"=w358) -> ("error out"=w355:errorcluster, "Instrument out"=w357:refnum<class "Instrument.lvclass">)  [unwired: 7 in]
          n145 = call "Write Instrument.lvclass.vi"("error in (no error)"=w355, "Instrument.lvclass"=w357, "S4ACS_GUI in"=w356) -> ("error out"=w352:errorcluster, "S4ACS_GUI out"=w341:refnum<class "S4GUI.lvclass">)  [unwired: 7 in]
          n146 = Bundle By Name(cluster=w341, "Obs_state"=w339) -> (w338:refnum<class "S4GUI.lvclass">)
        }
        frame 205 {
          # "Espera terminar a execução do comando atual \nantes de ir ao proximo passo da Observação."
          n147 = call "Read Instrument.lvclass.vi"("error in (no error)"=w378, "S4ACS_GUI in"=w379) -> ("error out"=w384:errorcluster, "Instrument.lvclass"=w385:refnum<class "Instrument.lvclass">, "S4ACS_GUI out"=w381:refnum<class "S4GUI.lvclass">)  [unwired: 7 in]
          n148 = call "Read WPSEL.vi"("error in (no error)"=w384, "Instrument in"=w385) -> ("error out"=w372:errorcluster, "Opt_Selector.lvclass"=w371:refnum<class "Opt_Selector.lvclass">, "Instrument out"=w383:refnum<class "Instrument.lvclass">)  [unwired: 7 in]
          n149 = call-dynamic "Read State Machine.vi"("error in (no error)"=w372, "Device in"=w371) -> ("error out"=w375:errorcluster, "State Machine.lvclass"=w376:refnum<class "State Machine.lvclass">, "Device out"=w369:refnum<class "Opt_Selector.lvclass">)  [unwired: 7 in]
          n150 = Increment(x=w362) -> (x+1=w361:u32)
          n151 = call-dynamic "Read State.vi"("error in (no error)"=w375, "State Machine in"=w376) -> ("error out"=w374:errorcluster, "State"=w364:i32, "State Machine out"=w373:refnum<class "State Machine.lvclass">)  [unwired: 7 in]
          n152 = Equal To 0?(x=w364) -> (x = 0?=w365:bool)
          n153 = call-dynamic "Write State Machine.vi"("error in (no error)"=w374, "State Machine.lvclass"=w373, "Device in"=w369) -> ("error out"=w368:errorcluster, "Device out"=w370:refnum<class "Opt_Selector.lvclass">)  [unwired: 7 in]
          n154 = call "Write WPSEL.vi"("error in (no error)"=w368, "Opt_Selector.lvclass"=w370, "Instrument in"=w383) -> ("error out"=w380:errorcluster, "Instrument out"=w382:refnum<class "Instrument.lvclass">)  [unwired: 7 in]
          n155 = Select(t=w361, s=w365, f=w362) -> (s? t:f=w363:u32)
          n156 = call "Write Instrument.lvclass.vi"("error in (no error)"=w380, "Instrument.lvclass"=w382, "S4ACS_GUI in"=w381) -> ("error out"=w377:errorcluster, "S4ACS_GUI out"=w367:refnum<class "S4GUI.lvclass">)  [unwired: 7 in]
          n157 = Bundle By Name(cluster=w367, "Obs_state"=w363) -> (w366:refnum<class "S4GUI.lvclass">)
        }
        frame 206 {
          # "Dispara o comando para o dispositivo corrente."
          n158 = call "Read Instrument.lvclass.vi"("error in (no error)"=w400, "S4ACS_GUI in"=w401) -> ("error out"=w406:errorcluster, "Instrument.lvclass"=w407:refnum<class "Instrument.lvclass">, "S4ACS_GUI out"=w403:refnum<class "S4GUI.lvclass">)  [unwired: 7 in]
          n159 = call "Read WPSEL.vi"("error in (no error)"=w406, "Instrument in"=w407) -> ("error out"=w394:errorcluster, "Opt_Selector.lvclass"=w395:refnum<class "Opt_Selector.lvclass">, "Instrument out"=w405:refnum<class "Instrument.lvclass">)  [unwired: 7 in]
          n160 = call "Read target name.vi"("error in (no error)"=w394, "Optics in"=w395) -> ("error out"=w388:errorcluster, "target name"=w393:string, "Optics out"=w387:refnum<class "Opt_Selector.lvclass">)  [unwired: 7 in]
          n161 = Equal?(x=w393, y="OFF") -> (x = y?=w391:bool)
          n162 = Increment(x=w397) -> (x+1=w389:u32)
          n163 = call "Write WPSEL.vi"("error in (no error)"=w388, "Opt_Selector.lvclass"=w387, "Instrument in"=w405) -> ("error out"=w402:errorcluster, "Instrument out"=w404:refnum<class "Instrument.lvclass">)  [unwired: 7 in]
          n164 = Select(t=u32 0, s=w391, f=w389) -> (s? t:f=w386:u32)
          n165 = call "Write Instrument.lvclass.vi"("error in (no error)"=w402, "Instrument.lvclass"=w404, "S4ACS_GUI in"=w403) -> ("error out"=w399:errorcluster, "S4ACS_GUI out"=w398:refnum<class "S4GUI.lvclass">)  [unwired: 7 in]
          n166 = Bundle By Name(cluster=w398, "Obs_state"=w386) -> (w396:refnum<class "S4GUI.lvclass">)
        }
        frame 207 {
          # "Dispara o comando para o dispositivo corrente."
          n167 = call "Read Instrument.lvclass.vi"("error in (no error)"=w423, "S4ACS_GUI in"=w424) -> ("error out"=w429:errorcluster, "Instrument.lvclass"=w430:refnum<class "Instrument.lvclass">, "S4ACS_GUI out"=w426:refnum<class "S4GUI.lvclass">)  [unwired: 7 in]
          n168 = call "Read WPROT.vi"("error in (no error)"=w429, "Instrument in"=w430) -> ("error out"=w416:errorcluster, "Opt_Selector.lvclass"=w415:refnum<class "Opt_Selector.lvclass">, "Instrument out"=w428:refnum<class "Instrument.lvclass">)  [unwired: 7 in]
          n169 = call-dynamic "Read State Machine.vi"("error in (no error)"=w416, "Device in"=w415) -> ("error out"=w419:errorcluster, "State Machine.lvclass"=w421:refnum<class "State Machine.lvclass">, "Device out"=w413:refnum<class "Opt_Selector.lvclass">)  [unwired: 7 in]
          n170 = call "Next State.vi"("error in (no error)"=w419, "New_State"=1, "State Machine in"=w421) -> ("error out"=w418:errorcluster, "State Machine out"=w417:refnum<class "State Machine.lvclass">)  [unwired: 7 in]
          n171 = call-dynamic "Write State Machine.vi"("error in (no error)"=w418, "State Machine.lvclass"=w417, "Device in"=w413) -> ("error out"=w412:errorcluster, "Device out"=w414:refnum<class "Opt_Selector.lvclass">)  [unwired: 7 in]
          n172 = Increment(x=w410) -> (x+1=w409:u32)
          n173 = call "Write WPROT.vi"("error in (no error)"=w412, "Opt_Selector.lvclass"=w414, "Instrument in"=w428) -> ("error out"=w425:errorcluster, "Instrument out"=w427:refnum<class "Instrument.lvclass">)  [unwired: 7 in]
          n174 = call "Write Instrument.lvclass.vi"("error in (no error)"=w425, "Instrument.lvclass"=w427, "S4ACS_GUI in"=w426) -> ("error out"=w422:errorcluster, "S4ACS_GUI out"=w411:refnum<class "S4GUI.lvclass">)  [unwired: 7 in]
          n175 = Bundle By Name(cluster=w411, "Obs_state"=w409) -> (w408:refnum<class "S4GUI.lvclass">)
        }
        frame 208 {
          # "Espera terminar a execução do comando atual \nantes de ir ao proximo passo da Observação."
          n176 = call "Read Instrument.lvclass.vi"("error in (no error)"=w448, "S4ACS_GUI in"=w449) -> ("error out"=w454:errorcluster, "Instrument.lvclass"=w455:refnum<class "Instrument.lvclass">, "S4ACS_GUI out"=w451:refnum<class "S4GUI.lvclass">)  [unwired: 7 in]
          n177 = call "Read WPROT.vi"("error in (no error)"=w454, "Instrument in"=w455) -> ("error out"=w442:errorcluster, "Opt_Selector.lvclass"=w441:refnum<class "Opt_Selector.lvclass">, "Instrument out"=w453:refnum<class "Instrument.lvclass">)  [unwired: 7 in]
          n178 = call-dynamic "Read State Machine.vi"("error in (no error)"=w442, "Device in"=w441) -> ("error out"=w445:errorcluster, "State Machine.lvclass"=w446:refnum<class "State Machine.lvclass">, "Device out"=w439:refnum<class "Opt_Selector.lvclass">)  [unwired: 7 in]
          n179 = call-dynamic "Read State.vi"("error in (no error)"=w445, "State Machine in"=w446) -> ("error out"=w444:errorcluster, "State"=w434:i32, "State Machine out"=w443:refnum<class "State Machine.lvclass">)  [unwired: 7 in]
          n180 = Equal To 0?(x=w434) -> (x = 0?=w435:bool)
          n181 = call-dynamic "Write State Machine.vi"("error in (no error)"=w444, "State Machine.lvclass"=w443, "Device in"=w439) -> ("error out"=w438:errorcluster, "Device out"=w440:refnum<class "Opt_Selector.lvclass">)  [unwired: 7 in]
          n182 = call "Write WPSEL.vi"("error in (no error)"=w438, "Opt_Selector.lvclass"=w440, "Instrument in"=w453) -> ("error out"=w450:errorcluster, "Instrument out"=w452:refnum<class "Instrument.lvclass">)  [unwired: 7 in]
          n183 = Select(t=u32 0, s=w435, f=w432) -> (s? t:f=w433:u32)
          n184 = call "Write Instrument.lvclass.vi"("error in (no error)"=w450, "Instrument.lvclass"=w452, "S4ACS_GUI in"=w451) -> ("error out"=w447:errorcluster, "S4ACS_GUI out"=w437:refnum<class "S4GUI.lvclass">)  [unwired: 7 in]
          n185 = Bundle By Name(cluster=w437, "Obs_state"=w433) -> (w436:refnum<class "S4GUI.lvclass">)
        }
        frame 220 {
          # "estado 30:\nmonta comando INIT"
          n186 = call "Read Instrument.lvclass.vi"("error in (no error)"=w502, "S4ACS_GUI in"=w503) -> ("error out"=w468:errorcluster, "Instrument.lvclass"=w469:refnum<class "Instrument.lvclass">, "S4ACS_GUI out"=w504:refnum<class "S4GUI.lvclass">)  [unwired: 7 in]
          n187 = call "Read WPSEL.vi"("error in (no error)"=w468, "Instrument in"=w469) -> ("error out"=w488:errorcluster, "Opt_Selector.lvclass"=w489:refnum<class "Opt_Selector.lvclass">, "Instrument out"=w496:refnum<class "Instrument.lvclass">)  [unwired: 7 in]
          n188 = call-dynamic "Read State Machine.vi"("error in (no error)"=w488, "Device in"=w489) -> ("error out"=w491:errorcluster, "State Machine.lvclass"=w493:refnum<class "State Machine.lvclass">, "Device out"=w490:refnum<class "Opt_Selector.lvclass">)  [unwired: 7 in]
          n189 = call "Next State.vi"("error in (no error)"=w491, "New_State"=30, "State Machine in"=w493) -> ("error out"=w460:errorcluster, "State Machine out"=w461:refnum<class "State Machine.lvclass">)  [unwired: 7 in]
          n190 = call-dynamic "Write State Machine.vi"("error in (no error)"=w460, "State Machine.lvclass"=w461, "Device in"=w490) -> ("error out"=w495:errorcluster, "Device out"=w497:refnum<class "Opt_Selector.lvclass">)  [unwired: 7 in]
          n191 = Increment(x=w494) -> (x+1=w499:u32)
          n192 = call "Write WPSEL.vi"("error in (no error)"=w495, "Opt_Selector.lvclass"=w497, "Instrument in"=w496) -> ("error out"=w466:errorcluster, "Instrument out"=w467:refnum<class "Instrument.lvclass">)  [unwired: 7 in]
          n193 = call "Read CALW.vi"("error in (no error)"=w466, "Instrument in"=w467) -> ("error out"=w479:errorcluster, "Opt_Selector.lvclass"=w480:refnum<class "Opt_Selector.lvclass">, "Instrument out"=w486:refnum<class "Instrument.lvclass">)  [unwired: 7 in]
          n194 = call-dynamic "Read State Machine.vi"("error in (no error)"=w479, "Device in"=w480) -> ("error out"=w482:errorcluster, "State Machine.lvclass"=w484:refnum<class "State Machine.lvclass">, "Device out"=w481:refnum<class "Opt_Selector.lvclass">)  [unwired: 7 in]
          n195 = call "Next State.vi"("error in (no error)"=w482, "New_State"=30, "State Machine in"=w484) -> ("error out"=w458:errorcluster, "State Machine out"=w459:refnum<class "State Machine.lvclass">)  [unwired: 7 in]
          n196 = call-dynamic "Write State Machine.vi"("error in (no error)"=w458, "State Machine.lvclass"=w459, "Device in"=w481) -> ("error out"=w485:errorcluster, "Device out"=w487:refnum<class "Opt_Selector.lvclass">)  [unwired: 7 in]
          n197 = call "Write CALW.vi"("error in (no error)"=w485, "Opt_Selector.lvclass"=w487, "Instrument in"=w486) -> ("error out"=w464:errorcluster, "Instrument out"=w465:refnum<class "Instrument.lvclass">)  [unwired: 7 in]
          n198 = call "Read GFOC.vi"("error in (no error)"=w464, "Instrument in"=w465) -> ("error out"=w470:errorcluster, "Opt_Continuous.lvclass"=w471:refnum<class "Opt_Continuous.lvclass">, "Instrument out"=w477:refnum<class "Instrument.lvclass">)  [unwired: 7 in]
          n199 = call-dynamic "Read State Machine.vi"("error in (no error)"=w470, "Device in"=w471) -> ("error out"=w473:errorcluster, "State Machine.lvclass"=w475:refnum<class "State Machine.lvclass">, "Device out"=w472:refnum<class "Opt_Continuous.lvclass">)  [unwired: 7 in]
          n200 = call "Next State.vi"("error in (no error)"=w473, "New_State"=30, "State Machine in"=w475) -> ("error out"=w456:errorcluster, "State Machine out"=w457:refnum<class "State Machine.lvclass">)  [unwired: 7 in]
          n201 = call-dynamic "Write State Machine.vi"("error in (no error)"=w456, "State Machine.lvclass"=w457, "Device in"=w472) -> ("error out"=w476:errorcluster, "Device out"=w478:refnum<class "Opt_Continuous.lvclass">)  [unwired: 7 in]
          n202 = call "Write GFOC.vi"("error in (no error)"=w476, "Opt_Continuous.lvclass"=w478, "Instrument in"=w477) -> ("error out"=w463:errorcluster, "Instrument out"=w462:refnum<class "Instrument.lvclass">)  [unwired: 7 in]
          n203 = call "Write Instrument.lvclass.vi"("error in (no error)"=w463, "Instrument.lvclass"=w462, "S4ACS_GUI in"=w504) -> ("error out"=w501:errorcluster, "S4ACS_GUI out"=w500:refnum<class "S4GUI.lvclass">)  [unwired: 7 in]
          n204 = Bundle By Name(cluster=w500, "Obs_state"=w499) -> (w498:refnum<class "S4GUI.lvclass">)
        }
        frame 221 {
          # "Espera terminar o homing de WPSEL,CALW e GMIR\nantes de seguir para o próximo estado."
          n205 = call "Read Instrument.lvclass.vi"("error in (no error)"=w533, "S4ACS_GUI in"=w534) -> ("error out"=w515:errorcluster, "Instrument.lvclass"=w516:refnum<class "Instrument.lvclass">, "S4ACS_GUI out"=w524:refnum<class "S4GUI.lvclass">)  [unwired: 7 in]
          n206 = call "Read CALW.vi"("error in (no error)"=w515, "Instrument in"=w516) -> ("error out"=w520:errorcluster, "Opt_Selector.lvclass"=w506:refnum<class "Opt_Selector.lvclass">)  [unwired: 7 in, 1 out]
          n207 = call "Read GFOC.vi"("error in (no error)"=w515, "Instrument in"=w516) -> ("error out"=w517:errorcluster, "Opt_Continuous.lvclass"=w505:refnum<class "Opt_Continuous.lvclass">)  [unwired: 7 in, 1 out]
          n208 = call "Read WPSEL.vi"("error in (no error)"=w515, "Instrument in"=w516) -> ("error out"=w530:errorcluster, "Opt_Selector.lvclass"=w529:refnum<class "Opt_Selector.lvclass">)  [unwired: 7 in, 1 out]
          n209 = call-dynamic "Read State Machine.vi"("error in (no error)"=w520, "Device in"=w506) -> ("error out"=w521:errorcluster, "State Machine.lvclass"=w522:refnum<class "State Machine.lvclass">)  [unwired: 7 in, 1 out]
          n210 = call-dynamic "Read State Machine.vi"("error in (no error)"=w517, "Device in"=w505) -> ("error out"=w518:errorcluster, "State Machine.lvclass"=w519:refnum<class "State Machine.lvclass">)  [unwired: 7 in, 1 out]
          n211 = call-dynamic "Read State Machine.vi"("error in (no error)"=w530, "Device in"=w529) -> ("error out"=w531:errorcluster, "State Machine.lvclass"=w532:refnum<class "State Machine.lvclass">)  [unwired: 7 in, 1 out]
          n212 = Increment(x=w526) -> (x+1=w525:u32)
          n213 = call-dynamic "Read State.vi"("error in (no error)"=w521, "State Machine in"=w522) -> ("error out"=w509:errorcluster, "State"=w513:i32)  [unwired: 7 in, 1 out]
          n214 = call-dynamic "Read State.vi"("error in (no error)"=w518, "State Machine in"=w519) -> ("error out"=w508:errorcluster, "State"=w512:i32)  [unwired: 7 in, 1 out]
          n215 = call-dynamic "Read State.vi"("error in (no error)"=w531, "State Machine in"=w532) -> ("error out"=w523:errorcluster, "State"=w514:i32)  [unwired: 7 in, 1 out]
          n216 = Compound Arithmetic op=ADD(w514, w513, w512) -> (w511:i32)
          n217 = Equal To 0?(x=w511) -> (x = 0?=w510:bool)
          n218 = Merge Errors(w523, w509, w508) -> (w507:errorcluster)
          n219 = Select(t=w525, s=w510, f=w526) -> (s? t:f=w527:u32)
          n220 = Bundle By Name(cluster=w524, "Obs_state"=w527) -> (w528:refnum<class "S4GUI.lvclass">)
        }
        frame 222 {
          n221 = call "Read Instrument.lvclass.vi"("error in (no error)"=w570, "S4ACS_GUI in"=w571) -> ("error out"=w541:errorcluster, "Instrument.lvclass"=w542:refnum<class "Instrument.lvclass">, "S4ACS_GUI out"=w572:refnum<class "S4GUI.lvclass">)  [unwired: 7 in]
